vi "AIT 1553 - ReadWrite Top Level.vi"(5 "Late?":bool, 6 "Iteration":i32, 7 "Mode":T17, 8 "error in (no error)":errorcluster, 9 "Iteration Duration":i64, 10 "Bus Section":T1, 11 "RT Data in":T2 {"Acyclic Frame Refs" format="%.0x"; "Label Transfer Config"."Block Data Refs"."Data Reference" format="%.0x"; "Status Config"."HWOut Dur Ref" format="%.0x"; "Status Config"."HWIn Dur Ref" format="%.0x"; "Status Config"."HWOut Count Ref" format="%.0x"; "Status Config"."HWIn Count Ref" format="%.0x"; "Status Config"."Error Data Ref" format="%.0x"; "HWOutput Channels"."Message Settings"."Driver Data"."First Word" min=8 max=31; "HWOutput Channels"."Message Settings"."Driver Data"."Num Bits" min=1 max=32; "HWOutput Channels"."Message Settings"."Driver Data"."Start Bit" min=8 max=31; "HWOutput Channels"."Message Settings"."Block Data Refs"."Data Reference" format="%.0x"; "HWInput Channels"."Message Settings"."Driver Data"."First Word" min=8 max=31; "HWInput Channels"."Message Settings"."Driver Data"."Num Bits" min=1 max=32; "HWInput Channels"."Message Settings"."Driver Data"."Start Bit" min=8 max=31; "HWInput Channels"."Message Settings"."Block Data Refs"."Data Reference" format="%.0x"}) -> (0 "error out":errorcluster, 3 "RT Data out":T2 {"Acyclic Frame Refs" format="%.0x"; "Label Transfer Config"."Block Data Refs"."Data Reference" format="%.0x"; "Status Config"."HWOut Dur Ref" format="%.0x"; "Status Config"."HWIn Dur Ref" format="%.0x"; "Status Config"."HWOut Count Ref" format="%.0x"; "Status Config"."HWIn Count Ref" format="%.0x"; "Status Config"."Error Data Ref" format="%.0x"; "HWOutput Channels"."Message Settings"."Driver Data"."First Word" min=8 max=31; "HWOutput Channels"."Message Settings"."Driver Data"."Num Bits" min=1 max=32; "HWOutput Channels"."Message Settings"."Driver Data"."Start Bit" min=8 max=31; "HWOutput Channels"."Message Settings"."Block Data Refs"."Data Reference" format="%.0x"; "HWInput Channels"."Message Settings"."Driver Data"."First Word" min=8 max=31; "HWInput Channels"."Message Settings"."Driver Data"."Num Bits" min=1 max=32; "HWInput Channels"."Message Settings"."Driver Data"."Start Bit" min=8 max=31; "HWInput Channels"."Message Settings"."Block Data Refs"."Data Reference" format="%.0x"})   [LabVIEW 2013, in "AIT 1553 Custom Device.lvlib"]
uses:
  AIT 1553 Custom Device.lvlib
  RT Controls/ReadWrite Selector.ctl
  RT Controls/AIT 1553  - RT Data.ctl
  RT Controls/AIT 1553 - RT HW Channel.ctl
  RT Controls/AIT 1553 - Bus Section.ctl
  RT Controls/AIT 1553 - RT Message Settings.ctl
  <vilib>/NI Veristand/Custom Device API/Block Data Reference.ctl
  <vilib>/NI Veristand/Custom Device API/Data Reference.ctl
  RT Controls/AIT 1553 - Driver Data.ctl
  Controls and Global/Start Bit.ctl
  Controls and Global/Number of Bits.ctl
  RT Controls/AIT 1553 - Board Config Info.ctl
  RT Controls/AIT 1553 - Hardware Type.ctl
  RT Controls/Error Qs.ctl
  RT Controls/Status Channels Config.ctl
  RT Controls/FIFO.ctl
  RT Controls/Label Transfer Config.ctl
  <vilib>/NI Veristand/Custom Device API/Custom Device Item Ref.ctl
  <vilib>/NI Veristand/Custom Device API/Custom Device API.lvlib
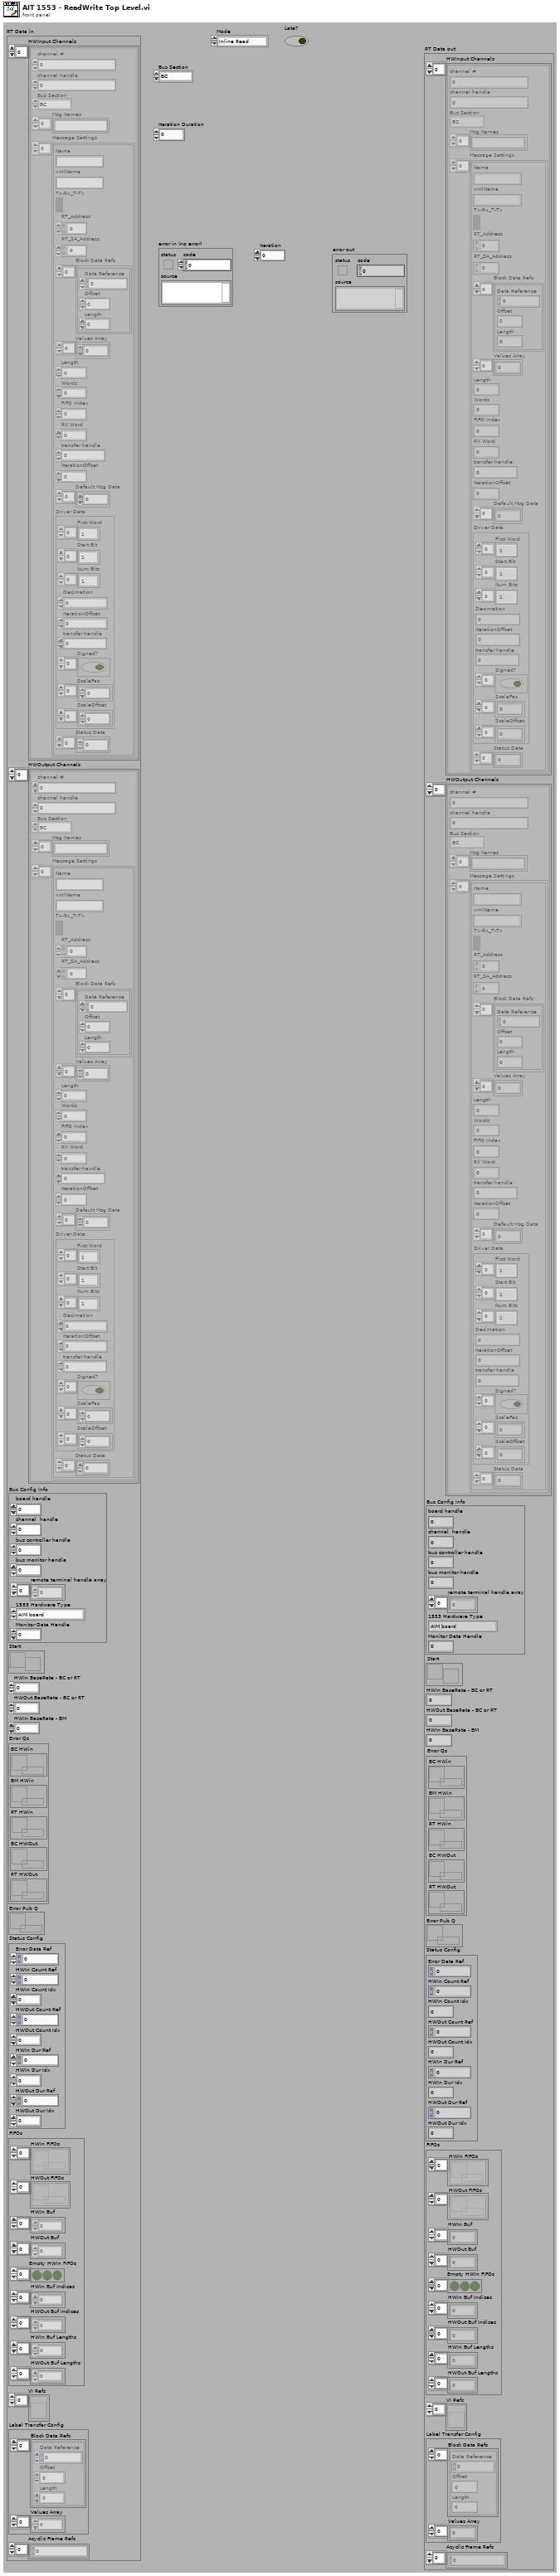
[diagram p1: front panel]
types:
  T1 = typedef "AIT 1553 Custom Device.lvlib/AIT 1553 - Bus Section.ctl" = enum16{"BC", "BM", "RT"}
  T2 = typedef "AIT 1553 Custom Device.lvlib/AIT 1553  - RT Data.ctl" = cluster{"HWInput Channels":T3[], "HWOutput Channels":T3[], "Bus Config Info":T10, "Start":refnum<notifier>, "HWIn BaseRate - BC or RT":i64, "HWOut BaseRate - BC or RT":i64, "HWIn BaseRate - BM":i64, "Error Qs":T12, "Error Pub Q":refnum<queue>, "Status Config":T13, "FIFOs":T14, "VI Refs":refnum<vi>[], "Label Transfer Config":T15, "Acyclic Frame Refs":T16[]}
  T3 = typedef "AIT 1553 Custom Device.lvlib/AIT 1553 - RT HW Channel.ctl" = cluster{"channel #":u16, "channel handle":u32, "Bus Section":T1, "Msg Names":string[], "Message Settings":T4[]}
  T4 = typedef "AIT 1553 Custom Device.lvlib/AIT 1553 - RT Message Settings.ctl" = cluster{"Name":string, "xmlName":string, "Tx-Rx_T-Tx":bool, "RT_Address":u8, "RT_SA_Address":u8, "Block Data Refs":T5[], "Values Array":dbl[], "Length":i32, "Words":i32, "FIFO Index":i32, "RX Word":u32, "transfer handle":u32, "IterationOffset":i32, "Default Msg Data":u16[], "Driver Data":T7, "Status Data":u32[]}
  T5 = typedef "Custom Device API.lvlib/Block Data Reference.ctl" = cluster{"Data Reference":T6, "Offset":i32, "Length":i32}
  T6 = typedef "Custom Device API.lvlib/Data Reference.ctl" = i32
  T7 = typedef "AIT 1553 Custom Device.lvlib/AIT 1553 - Driver Data.ctl" = cluster{"First Word":T8[], "Start Bit":T8[], "Num Bits":T9[], "Decimation":i32, "IterationOffset":i32, "transfer handle":u32, "Signed?":bool[], "ScaleFac":dbl[], "ScaleOffset":dbl[]}
  T8 = typedef "AIT 1553 Custom Device.lvlib/Start Bit.ctl" = i32
  T9 = typedef "AIT 1553 Custom Device.lvlib/Number of Bits.ctl" = i32
  T10 = typedef "AIT 1553 Custom Device.lvlib/AIT 1553 - Board Config Info.ctl" = cluster{"board handle":u32, "channel  handle":u32, "bus controller handle":u32, "bus monitor handle":u32, "remote terminal handle array":u32[], "1553 Hardware Type":T11, "Monitor Data Handle":u32}
  T11 = typedef "AIT 1553 Custom Device.lvlib/AIT 1553 - Hardware Type.ctl" = enum16{"AIM board", "AIT Board"}
  T12 = typedef "AIT 1553 Custom Device.lvlib/Error Qs.ctl" = cluster{"BC HWin":refnum<queue>, "BM HWin":refnum<queue>, "RT HWin":refnum<queue>, "BC HWOut":refnum<queue>, "RT HWOut":refnum<queue>}
  T13 = typedef "AIT 1553 Custom Device.lvlib/Status Channels Config.ctl" = cluster{"Error Data Ref":T6, "HWIn Count Ref":T6, "HWIn Count Idx":i32, "HWOut Count Ref":T6, "HWOut Count Idx":i32, "HWIn Dur Ref":T6, "HWIn Dur Idx":i32, "HWOut Dur Ref":T6, "HWOut Dur Idx":i32}
  T14 = typedef "AIT 1553 Custom Device.lvlib/FIFO.ctl" = cluster{"HWIn FIFOs":refnum<k33>[], "HWOut FIFOs":refnum<k33>[], "HWIn Buf":dbl[], "HWOut Buf":dbl[], "Empty HWIn FIFOs":bool[], "HWIn Buf Indices":i32[], "HWOut Buf Indices":i32[], "HWIn Buf Lengths":i32[], "HWOut Buf Lengths":i32[]}
  T15 = typedef "AIT 1553 Custom Device.lvlib/Label Transfer Config.ctl" = cluster{"Block Data Refs":T5[], "Values Array":dbl[]}
  T16 = typedef "Custom Device API.lvlib/Custom Device Item Ref.ctl" = u64
  T17 = typedef "AIT 1553 Custom Device.lvlib/ReadWrite Selector.ctl" = enum16{"Inline Read", "Inline Write", "Async HWIn", "Async HWOut"}
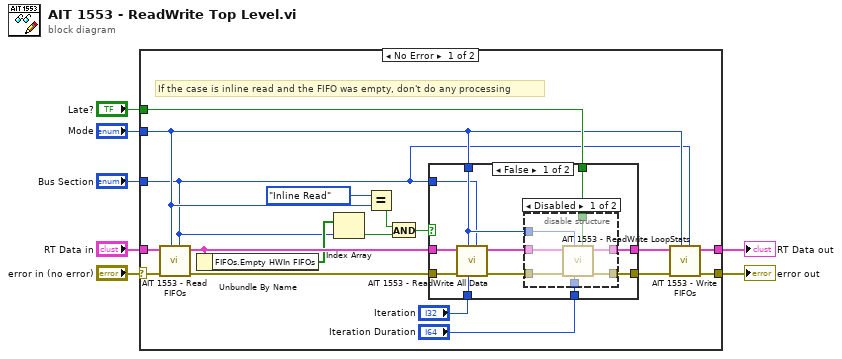
[diagram p0: block diagram]
diagram:
  n1 = case shown="No Error" "error in (no error)" {
    selector: "error in (no error)" -> [w18 w49]
    tunnel: "RT Data in" -> [w25 w48]
    tunnel: [w24 w48] -> w6
    tunnel: [w23 w49] -> w5
    tunnel: "Mode" -> [w11 _]
    tunnel: "Late?" -> [w13 _]
    tunnel: "Bus Section" -> [w9 _]
    frame No Error {
      # "If the case is inline read and the FIFO was empty, don't do any processing"
      n2 = call "AIT 1553 - Read FIFOs.vi"("Bus Section"=w9, "Mode"=w11, "error in (no error)"=w18, "RT Data in"=w25) -> ("error out"=w22:errorcluster, "RT Data out"=w14:T2)  [unwired: 6 in]
      n3 = Unbundle By Name(w14) -> ("FIFOs.Empty HWIn FIFOs"=w10:bool[])
      n4 = Index Array(array=w10, index=w9) -> (element=w8:bool)
      n5 = Equal?(x=ReadWrite_Selector."Inline Read", y=w11) -> (x = y?=w20:bool)
      n6 = And(x=w20, y=w8) -> (x .and. y?=w12:bool)
      n7 = case shown="False" w12 {
        tunnel: w22 -> [w36 w47]
        tunnel: [w31 w47] -> w16
        tunnel: [w30 w46] -> w15
        tunnel: w14 -> [w35 w46]
        tunnel: w11 -> [w27 _]
        tunnel: "Iteration" -> [w34 _]
        tunnel: w13 -> [w29 _]
        tunnel: "Iteration Duration" -> [w28 _]
        tunnel: w9 -> [w26 _]
        frame False {
          n8 = call "AIT 1553 - ReadWrite All Data.vi"("Bus Section"=w26, "Iteration"=w34, "Mode"=w27, "error in (no error)"=w36, "RT Data in"=w35) -> ("error out"=w32:errorcluster, "RT Data out"=w33:T2)  [unwired: 5 in]
          n9 = disable-structure shown="Disabled" {
            disable-tunnel: w33 -> [w43 w45]
            disable-tunnel: w32 -> [w42 w44]
            disable-tunnel: [w41 w44] -> w31
            disable-tunnel: [w40 w45] -> w30
            disable-tunnel: w29 -> [w39 _]
            disable-tunnel: w28 -> [w38 _]
            disable-tunnel: w27 -> [w37 _]
            frame Disabled {
              n10 = call "AIT 1553 - ReadWrite LoopStats.vi"("Late"=w39, "Iteration Duration"=w38, "Mode"=w37, "error in (no error)"=w42, "RT Data in"=w43) -> ("error out"=w41:errorcluster, "RT Data out"=w40:T2)  [unwired: 5 in]
            }
            frame Enabled {
            }
          }
        }
        frame True {
        }
      }
      n11 = call "AIT 1553 - Write FIFOs.vi"("Bus Section"=w9, "Mode"=w11, "error in (no error)"=w16, "RT Data in"=w15) -> ("error out"=w23:errorcluster, "RT Data out"=w24:T2)  [unwired: 6 in]
    }
    frame Error {
    }
  }
  "error out" <- w5
  "RT Data out" <- w6
